vi "SIM compute jacobian.vi"(6 "reset?":bool, 8 "Current jacobian":dbl[][](array[numeric]), 10 "F(y)":dbl[](array[numeric]) format="%.16e", 11 "y current":dbl[](array[numeric]) format="%.16e") -> (0 "Current jacobian out":dbl[][](array[numeric]), 1 "finished?":bool, 2 "F(y_0)":dbl[](array[numeric]) format="%.16f", 3 "y next":dbl[](array[numeric]) format="%.16f")   [LabVIEW 2017]
uses:
  <vilib>/Simulation/ContinuousLinear/Implementation/Shared/Solvers/SIM BDF.llb/SIM BDF jacobian stages.ctl
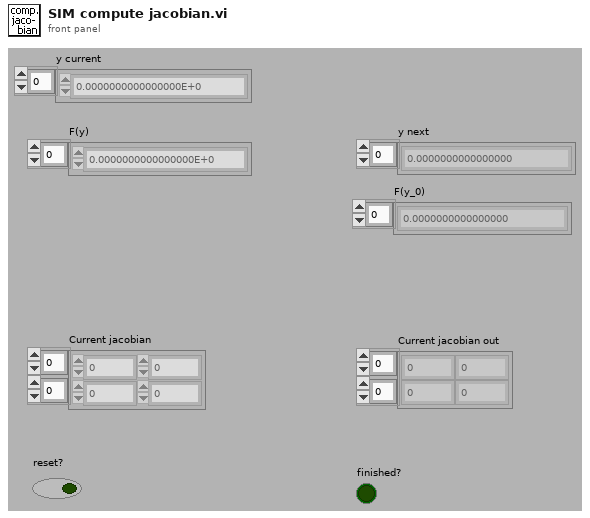
[diagram p1: front panel]
types:
  T1 = typedef "SIM BDF jacobian stages.ctl" = enum16{"first output", "second output"}
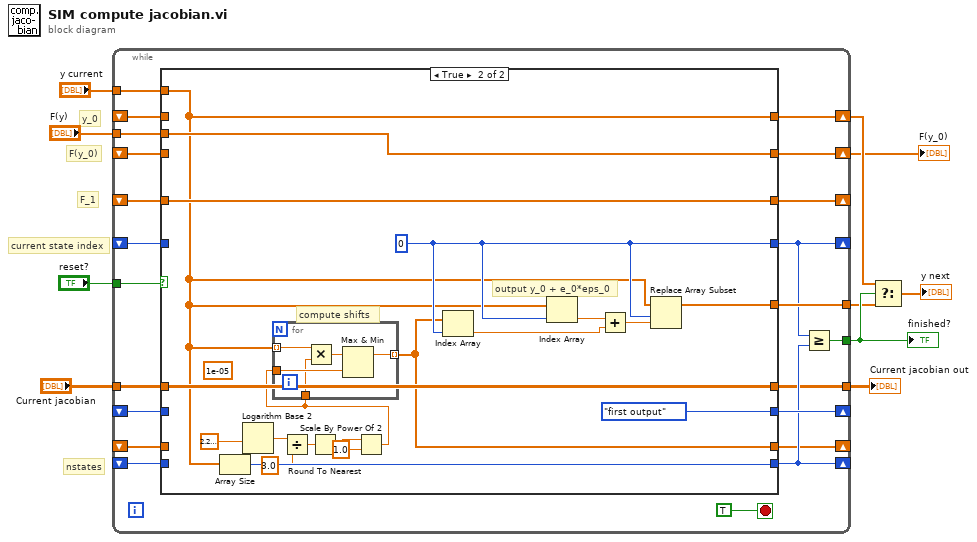
[diagram p0: block diagram]
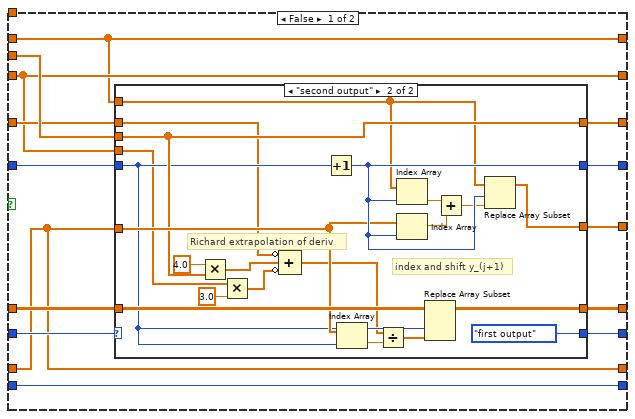
[diagram p2: hidden frame]
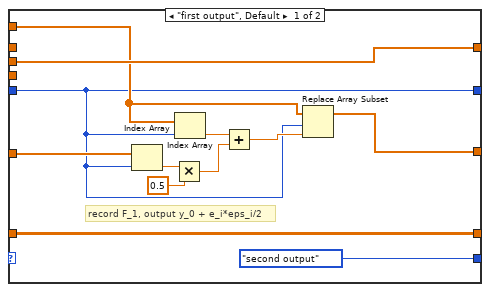
[diagram p3: hidden frame]
diagram:
  # "nstates"
  # "F_1"
  # "y_0"
  # "current state index"
  # "F(y_0)"
  n1 = while {
    tunnel: "reset?" -> [w31]
    shift-right: [w29] -> w1
    shift-left: _ -> [w28]
    tunnel: "F(y)" -> [w30]
    shift-right: [w15] -> _
    shift-left: _ -> [w19]
    shift-right: [w26] -> w3
    shift-left: _ -> [w25]
    tunnel: "y current" -> [w27]
    tunnel: [w23] -> w4
    shift-right: [w22] -> _
    shift-left: _ -> [w21]
    shift-right: [w20] -> _
    shift-left: _ -> [w18]
    shift-right: [w16] -> _
    shift-left: _ -> [w17]
    tunnel: [w14] -> w5
    tunnel: "Current jacobian" -> [w13]
    tunnel: [w12] -> w6
    shift-right: [w11] -> _
    shift-left: _ -> [w24]
    stop <- TRUE stop-if-true
    n2 = case shown="True" w31 {
      tunnel: w30 -> [w45 w98]
      tunnel: [w37 w98] -> w29
      tunnel: w28 -> [w37 _]
      tunnel: [w39 w94] -> w15
      tunnel: w27 -> [_ w88]
      tunnel: [w34 w88] -> w26
      tunnel: w25 -> [w34 _]
      tunnel: w24 -> [w33 _]
      tunnel: [w42 w93] -> w23
      tunnel: [w35 SIM_BDF_jacobian_stages."first output" ("Jacobian computation stage")] -> w22
      tunnel: w21 -> [w46 _]
      tunnel: [w44 w91] -> w20
      tunnel: w19 -> [w43 _]
      tunnel: w18 -> [w41 w91]
      tunnel: [w40 w89] -> w16
      tunnel: w17 -> [w40 _]
      tunnel: w13 -> [w38 w90]
      tunnel: [w36 w90] -> w12
      tunnel: [w33 w87] -> w11
      frame False {
        n3 = case shown="\"second output\"" w46 {
          tunnel: w45 -> [w58 w74]
          tunnel: [w58 w74] -> w44
          tunnel: w33 -> [w50 w76]
          tunnel: w43 -> [w48 w72]
          tunnel: w34 -> [w55 w59]
          tunnel: [w54 w73] -> w42
          tunnel: w41 -> [_ w70]
          tunnel: [w48 w79] -> w39
          tunnel: w38 -> [w47 w78]
          tunnel: w37 -> [_ w69]
          tunnel: [w47 w77] -> w36
          tunnel: [SIM_BDF_jacobian_stages."second output" ("Jacobian computation stage") SIM_BDF_jacobian_stages."first output" ("Jacobian computation stage")] -> w35
          frame "first output", Default {
            # "record F_1, output y_0 + e_i*eps_i/2"
            n4 = Index Array(array=w50, index=w48) -> (element=w53:dbl)
            n5 = Multiply(x=w53, y=0.5) -> (x*y=w51:dbl)
            n6 = Index Array(array=w55, index=w48) -> (element=w57:dbl)
            n7 = Add(x=w57, y=w51) -> (x+y=w56:dbl)
            n8 = Replace Array Subset(array=w55, new element=w56, index=w48) -> (w54:dbl[])
          }
          frame "second output" {
            # "Richard extrapolation of deriv"
            # "index and shift y_(j+1)"
            n9 = Multiply(x=4.0, y=w74) -> (x*y=w61:dbl[])
            n10 = Multiply(x=w69, y=3.0) -> (x*y=w63:dbl[])
            n11 = Compound Arithmetic op=ADD(invert w70, w61, invert w63) -> (w68:dbl[])
            n12 = Increment(x=w72) -> (x+1=w79:i32)
            n13 = Index Array(array=w76, index=w72) -> (element=w67:dbl)
            n14 = Divide(x=w68, y=w67) -> (x/y=w60:dbl[])
            n15 = Index Array(array=w59, index=w79) -> (element=w65:dbl)
            n16 = Index Array(array=w76, index=w79) -> (element=w66:dbl)
            n17 = Replace Array Subset(array=w78, new element=w60, index (col)=w72) -> (w77:dbl[][])  [unwired: 1 in]
            n18 = Add(x=w65, y=w66) -> (x+y=w64:dbl)
            n19 = Replace Array Subset(array=w59, new element=w64, index=w79) -> (w73:dbl[])
          }
        }
      }
      frame True {
        (unwired) 1e-05
        w94 = 0
        # "compute shifts"
        # "output y_0 + e_0*eps_0"
        n20 = Array Size(array=w88) -> (size(s)=w89:i32)
        n21 = Logarithm Base 2(1:2.220446049250313e-16) -> (0:w86:dbl)
        n22 = Divide(x=w86, y=3.0) -> (x/y=w84:dbl)
        n23 = Round To Nearest(number=w84) -> (nearest integer value=w83:dbl)
        n24 = Scale By Power Of 2(n=w83, x=1.0) -> (x*2^n=w81:dbl)
        n25 = for {
          tunnel: w81 -> [w103]
          tunnel: w88 -> [w101] mode=indexing
          tunnel: w81 -> [w102]
          tunnel: [w99] -> w87 mode=indexing
          n26 = Multiply(x=w101, y=w102) -> (x*y=w100:dbl)
          n27 = Max & Min(x=w100, y=w103) -> (max(x,y)=w99:dbl)  [unwired: 1 out]
        }
        n28 = Index Array(array=w87, index=w94) -> (element=w96:dbl)
        n29 = Index Array(array=w88, index=w94) -> (element=w97:dbl)
        n30 = Add(x=w97, y=w96) -> (x+y=w95:dbl)
        n31 = Replace Array Subset(array=w88, new element=w95, index=w94) -> (w93:dbl[])
      }
    }
    n32 = Greater Or Equal?(x=w15, y=w16) -> (x >= y?=w14:bool)
  }
  "finished?" <- w5
  "Current jacobian out" <- w6
  "F(y_0)" <- w1
  n33 = Select(t=w3, s=w5, f=w4) -> (s? t:f=→"y next":dbl[])
